vi "HFRR ADV v036 new software.vi"() -> ()   [LabVIEW 2025] (continued)
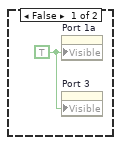
[diagram p5: hidden frame]
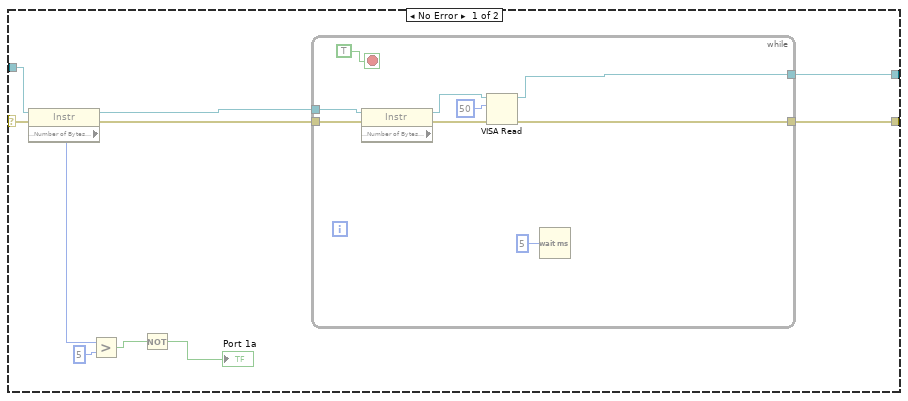
[diagram p6: hidden frame]
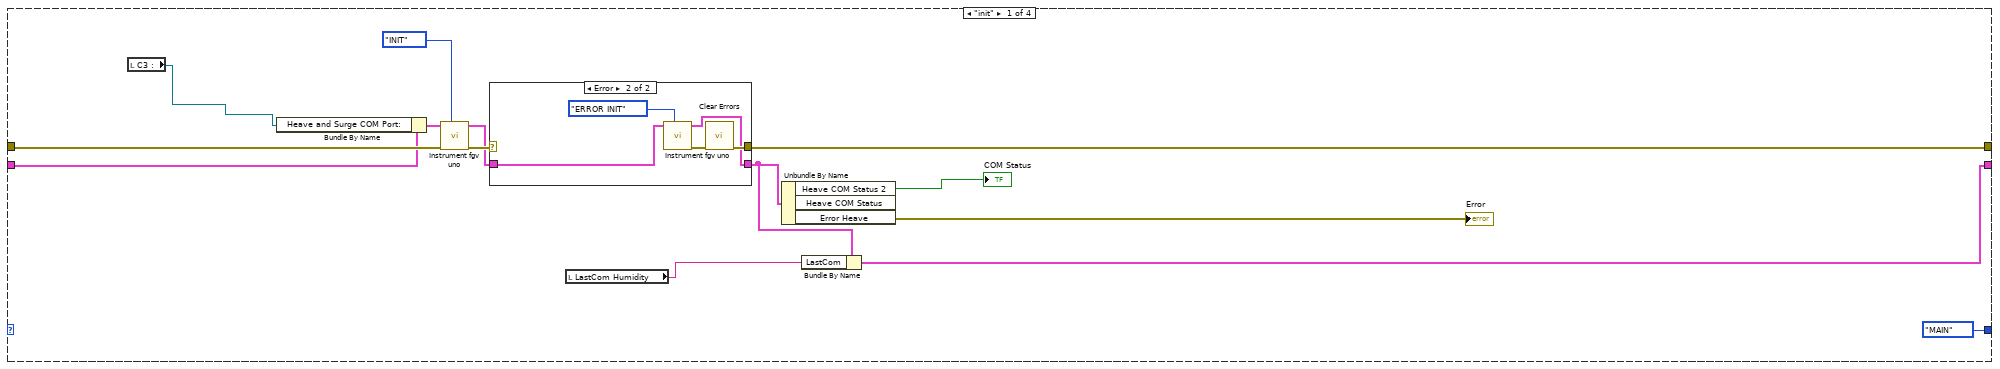
[diagram p8: hidden frame]
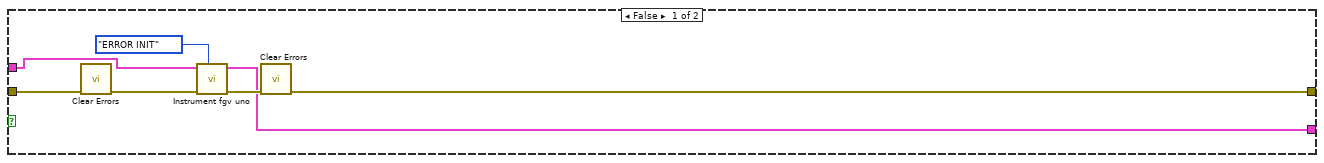
[diagram p10: hidden frame]
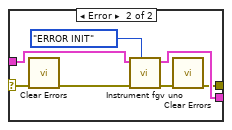
[diagram p12: hidden frame]
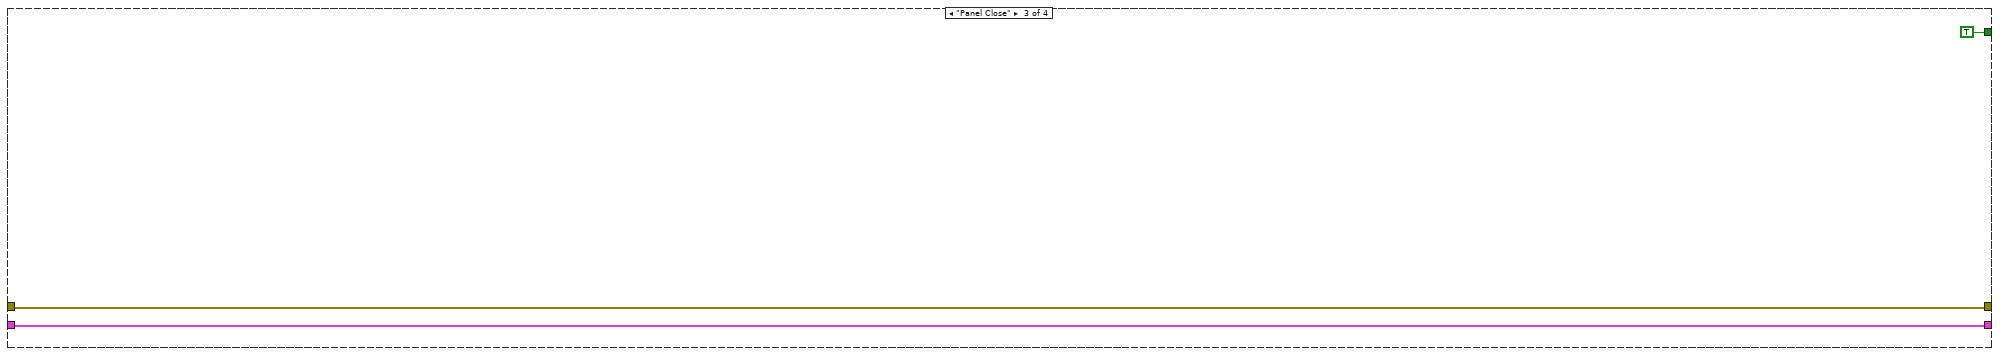
[diagram p14: hidden frame]
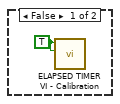
[diagram p18: hidden frame]
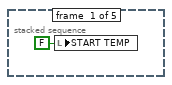
[diagram p20: hidden frame]
      frame Disabled {
        n3364 = local read "Read HUMIDITY"() -> (w4403:string)
        n3365 = Spreadsheet String To Array(delimiter (Tab)=",", format string="", spreadsheet string=w4403, array type (2D Dbl)=string[] []) -> (array=w4422:string[])
        n3366 = for {
          tunnel: w4422 -> [w4431] mode=indexing
          tunnel: string[] ["STATE;", "SET;", "RH;", "T;", "AMB_RH;", "AMB_T;", "PUMP;", "FAN_IN;", "FAN_OUT;", "DEHUM;", "CURRENT;", "STALL;"] -> [w4430] mode=indexing
          tunnel: [w4429] -> w4421 mode=indexing
          n3367 = Match Pattern(string=w4431, regular expression=w4430) -> (after substring=w4429:string)  [unwired: 1 in, 3 out]
        }
        n3368 = Index Array(array=w4421) -> (element #1=→"STATE :":string, element #2=→"SET :":string, element #3=w4411:string, element #4=→"T :":string, element #5=w4409:string, element #6=→"AMB_T :":string, element #7=→"PUMP :":string, element #8=→"FAN_IN :":string, element #9=→"FAN_OUT :":string, element #10=→"DEHUM :":string, element #11=→"CURRENT :":string, element #12=→"STALL :":string)  [unwired: 12 in]
        "RH :" <- w4411
        "AMB_RH :" <- w4409
        n3369 = Fract/Exp String To Number(string=w4411) -> (number=w4404:dbl)  [unwired: 3 in, 1 out]
        n3370 = Fract/Exp String To Number(string=w4409) -> (number=w4408:dbl)  [unwired: 3 in, 1 out]
        n3371 = local write "Ambient Humidity :"(w4408) -> ()
        n3372 = Equal?(x=w4404, y=0.0) -> (x = y?=w4406:bool)
        n3373 = case shown="True" w4406 {
          tunnel: [w4427 w4428] -> w4405
          tunnel: w4404 -> [w4427 _]
          frame False {
            (unwired) 0.0
            "Humidity temp" <- w4427
          }
          frame True {
            n3374 = local read "Humidity temp"() -> (w4428:dbl)
          }
        }
        "RH Numeric:" <- w4405
      }
      frame Enabled {
        n3375 = local read "Read HUMIDITY"() -> (w4454:string)
        n3376 = Spreadsheet String To Array(delimiter (Tab)=",", format string="", spreadsheet string=w4454, array type (2D Dbl)=dbl[] []) -> (array=w4450:dbl[])
        n3377 = Index Array(array=w4450) -> (element #1=→"STATE :":dbl, element #2=→"SET :":dbl, element #3=w4435:dbl, element #4=→"RH :":dbl, element #5=→"T :":dbl, element #6=→"AMB_RH :":dbl, element #7=→"AMB_T :":dbl, element #8=→"PUMP :":dbl, element #9=→"FAN_IN :":dbl, element #10=→"FAN_OUT :":dbl, element #11=→"DEHUM :":dbl, element #12=→"CURRENT :":dbl, element #13=→"STALL":dbl)  [unwired: 13 in]
        "RH Numeric:" <- w4435
        n3378 = Equal?(x=w4435, y=0.0) -> (x = y?=w4438:bool)
        n3379 = case shown="False" w4438 {
          tunnel: [w4455 w4456] -> w4434
          tunnel: w4435 -> [w4455 _]
          frame False {
            "Humidity temp 2" <- w4455
          }
          frame True {
            n3380 = local read "Humidity temp 2"() -> (w4456:dbl)
          }
        }
        n3381 = call <vilib>:"Median Filter PtByPt.vi"("rank"=2, "x"=w4434) -> ("Filtered x"=w4433:dbl)  [unwired: 2 in, 1 out]
      }
    }
    n3382 = local write "RH Numeric:"(w4400) -> ()
    n3383 = local read "Quit"() -> (w4402:bool)
  }
  n3384 = while {
    shift-right: [w4462] -> _
    shift-left: _ -> [w4463]
    shift-right: [w4460] -> _
    shift-left: T20 {"Read Uno"="", "Bytes at Heave Port"=0.0, "UNO COM Port:"="COM9", "UNO COM Port: 2"="COM7", "Residual Due"="", "UNO COM Status 2"=TRUE, "UNO COM Status"=TRUE, "Port 2"=TRUE, "Sway PPR"=6400.0, "Surge PPR"=6400.0, "Heave PPR"=6400.0, "Sway Pitch"=2.0, "Surge Pitch"=3.0, "Heave Pitch"=4.0, "Sway Pulses/mm"=320.0, "Surge Pulses/mm"=1600.0, "Heave Pulses/mm"=1600.0, "inner loop"=0.0, "Read Heave and Surge 2"="", "String 36"="", "Write S"=FALSE, "WriteCC1"=[""], "Heave COM Loop"=0, "LastCom"="", "EXIT"=FALSE, "Error Heave"={"status"=TRUE, "code"=-1073807343, "source"=""}} -> [w4459]
    shift-right: [w4457] -> _
    shift-left: enum16{"init", "MAIN", "Panel Close"}."init" -> [w4458]
    stop <- w4461 stop-if-true
    # "UNO CODE LOGIC"
    n3385 = case shown="\"MAIN\"" w4458 {
      tunnel: w4463 -> [w4477 w4496 w4552 w4554]
      tunnel: [w4472 w4501 w4552 w4554] -> w4462
      tunnel: [_ _ TRUE _] -> w4461
      tunnel: [w4468 w4499 w4550 w4553] -> w4460
      tunnel: w4459 -> [w4474 w4495 w4550 w4553]
      tunnel: [enum16{"init", "MAIN", "Panel Close"}."MAIN" w4490 _ _] -> w4457
      frame "init" {
        n3386 = local read "Com Port 1"() -> (w4464:refnum<visa-resource-name>)
        n3387 = Bundle By Name(cluster=w4474, "UNO COM Port:"=w4464) -> (w4473:T20)
        n3388 = call "Instrument fgv.vi"("Enum"=T31."INIT", "error in (no error) 2"=w4477, "INPUT"=w4473) -> ("error"=w4475:errorcluster, "output"=w4471:T18)  [unwired: 6 in, 1 out]
        n3389 = case shown="Error" w4475 {
          selector: w4475 -> [w4479 _]
          tunnel: [w4479 w4483] -> w4472
          tunnel: w4471 -> [w4478 w4481]
          tunnel: [w4478 w4480] -> w4469
          frame No Error {
          }
          frame Error {
            n3390 = call "Instrument fgv.vi"("Enum"=T31."ERROR INIT", "INPUT"=w4481) -> ("error"=w4484:errorcluster, "output"=w4480:T18)  [unwired: 7 in, 1 out]
            n3391 = call <vilib>:"Clear Errors.vi"("error in (no error)"=w4484) -> ("error out"=w4483:errorcluster)  [unwired: 5 in, 1 out]
          }
        }
        n3392 = local read "LastCom UNO"() -> (w4466:string)
        n3393 = Unbundle By Name(w4469) -> ("Heave COM Status 2"=→"Instrument Status":bool, "Error Heave"=→"Error  2":errorcluster)  [unwired: 1 out]
        n3394 = Bundle By Name(cluster=w4469, "LastCom"=w4466) -> (w4468:T18)
      }
      frame "MAIN" {
        n3395 = Unbundle By Name(w4495) -> ("UNO COM Port: 2"=w4485:refnum<visa-resource-name>)
        n3396 = local read "Com Port 1"() -> (w4486:refnum<visa-resource-name>)
        n3397 = local write "COM Port UNO :"(w4485) -> ()
        n3398 = Equal?(x=w4485, y=w4486) -> (x = y?=w4502:bool)
        n3399 = Bundle By Name(cluster=w4495, "UNO COM Port:"=w4486) -> (w4494:T20)
        n3400 = case shown="True" w4502 {
          tunnel: [w4506 w4523] -> w4501
          tunnel: w4496 -> [w4507 w4529]
          tunnel: w4494 -> [w4505 w4527]
          tunnel: [w4504 w4522] -> w4499
          frame False {
            n3401 = call <vilib>:"Clear Errors.vi"("error in (no error)"=w4507) -> ("error out"=w4503:errorcluster)  [unwired: 5 in, 1 out]
            n3402 = call "Instrument fgv.vi"("Enum"=T31."ERROR INIT", "error in (no error) 2"=w4503, "INPUT"=w4505) -> ("error"=w4509:errorcluster, "output"=w4504:T18)  [unwired: 6 in, 1 out]
            n3403 = call <vilib>:"Clear Errors.vi"("error in (no error)"=w4509) -> ("error out"=w4506:errorcluster)  [unwired: 5 in, 1 out]
          }
          frame True {
            n3404 = call "Instrument fgv.vi"("Enum"=T31."READ", "error in (no error) 2"=w4529, "INPUT"=w4527) -> ("error"=w4528:errorcluster, "output"=w4521:T18)  [unwired: 6 in, 1 out]
            n3405 = Bundle By Name(cluster=w4521, "String 36"="WRITE UNO") -> (w4520:T18)
            n3406 = case shown="True" "Write" {
              selector: "Write" -> [_ w4544]
              tunnel: w4528 -> [w4542 w4549]
              tunnel: [w4542 w4548] -> w4518
              tunnel: w4520 -> [w4541 w4546]
              tunnel: [w4541 w4545] -> w4517
              frame False {
              }
              frame True {
                n3407 = Not(x=w4544) -> (.not. x?=w4543:bool)
                n3408 = local write "Write"(w4543) -> ()
                n3409 = call "Instrument fgv.vi"("Enum"=T31."MANUAL WRITE", "error in (no error) 2"=w4549, "INPUT"=w4546) -> ("error"=w4548:errorcluster, "output"=w4545:T18)  [unwired: 6 in, 1 out]
              }
            }
            n3410 = Array Size(array="Write UNO") -> (size(s)=w4515:i32)
            n3411 = Greater Than 0?(x=w4515) -> (x > 0?=w4514:bool)
            n3412 = call "Instrument fgv.vi"("Enum"=T31."WRITE", "error in (no error) 2"=w4518, "WriteCC1"="Write UNO", "INPUT"=w4517) -> ("error"=w4525:errorcluster, "WriteCC1 2"=w4516:string[], "output"=w4524:T18)  [unwired: 5 in]
            n3413 = case shown="True" w4514 {
              tunnel: w4516 -> [_ w4531]
              frame False {
              }
              frame True {
                n3414 = local write "Write UNO"(w4531) -> ()
              }
            }
            n3415 = case shown="Error" w4525 {
              selector: w4525 -> [w4532 w4535]
              tunnel: w4524 -> [w4533 w4540]
              tunnel: [w4533 w4539] -> w4522
              tunnel: [w4532 w4537] -> w4523
              frame No Error {
              }
              frame Error {
                n3416 = call <vilib>:"Clear Errors.vi"("error in (no error)"=w4535) -> ("error out"=w4534:errorcluster)  [unwired: 5 in, 1 out]
                n3417 = call "Instrument fgv.vi"("Enum"=T31."ERROR INIT", "error in (no error) 2"=w4534, "INPUT"=w4540) -> ("error"=w4538:errorcluster, "output"=w4539:T18)  [unwired: 6 in, 1 out]
                n3418 = call <vilib>:"Clear Errors.vi"("error in (no error)"=w4538) -> ("error out"=w4537:errorcluster)  [unwired: 5 in, 1 out]
              }
            }
            n3419 = Unbundle By Name(w4522) -> ("LastCom"=→"LastCom UNO":string, "Read Heave and Surge"=→"Read UNO":string)
          }
        }
        n3420 = Unbundle By Name(w4499) -> ("Heave COM Status 2"=w4500:bool, "Heave COM Status"=w4489:bool, "Error Heave"=w4487:errorcluster, "Bytes at Heave Port"=→"Bytes at Humidity Port":dbl)
        n3421 = Not(x=w4489) -> (.not. x?=w4497:bool)
        n3422 = Not(x=w4500) -> (.not. x?=w4488:bool)
        n3423 = local write "Instrument Status"(w4497) -> ()
        n3424 = local write "Error  2"(w4487) -> ()
        n3425 = local write "Port 1a"(w4489) -> ()
        n3426 = local read "Quit"() -> (w4491:bool)
        n3427 = local write "COM Status"(w4488) -> ()
        n3428 = Select(t=enum16{"init", "MAIN", "Panel Close"}."Panel Close", s=w4491, f=enum16{"init", "MAIN", "Panel Close"}."MAIN") -> (s? t:f=w4490:enum16{"init", "MAIN", "Panel Close"})
      }
      frame "Panel Close" {
      }
      frame Default {
      }
    }
  }
